vi "CRYStart Editor.vi"(11 "Project Tree reference":refnum<vi>) -> (1 "Steps config.":bool[](array[boolean]))   [LabVIEW 2013]
uses:
  Typedef Control/CRYStart Cluster.ctl
panel:
  in  "Update Display during sequence":bool caption="在运行序列中更新显示步骤"
  in  "Clear measured data at start of sequence":bool caption="在序列开始时清除测试数据"
  in  "Close opened Display at start of sequence":bool caption="在序列开始时关闭打开显示步骤"
  in  "Preload Stimulus":bool caption="预加载激励"
  out "Step Name":string
  in  "Use same Calibration in all subsequences":bool caption="在所有的局部序列使用相同的校准"
  in  "Use same Hardware in all subsequences":bool caption="在所有的局部序列使用相同的硬件"
  in  "Halt on FAIL":bool caption="失败时中断"
  in  "Display for confirmation":bool caption="显示确认"
  in  "Cancel button":bool
  in  "OK button":bool
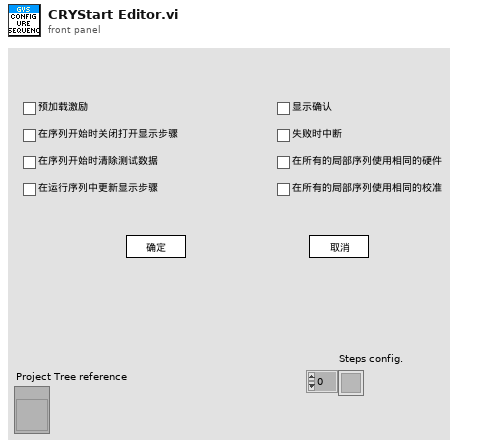
[diagram p1: front panel]
types:
  T1 = typedef "CRYStep.ctl" = cluster{"No.VI":i32, "Category":string, "StepName":string, "Seq setup flattened":string, "Comment":string, "Steps config.":bool[], "Jump config":i32[], "Start":dbl, "Increment":dbl, "Name":string, "Unit":string, "Y data":u16, "Y prefix":string, "Y dB ref":dbl, "Y unit":string, "Repeat State Array":cluster{"Start":dbl, "Increment":dbl, "Count":i32, "Num":i32}[]}
  T2 = typedef "CRYStart Cluster.ctl" = cluster{"SequenceName":string, "Preload Stimulus":bool, "CloseOpenedDisplay":bool, "ClearMeasuredData":bool, "UpdateDisplayDuringRun":bool, "DisplayForConfirmation":bool, "HaltOnFail":bool, "UseSameHardware":bool, "UseSameCalibration":bool}
  T3 = cluster{"SourceRowNum":i32, "SourceCount":i32, "TargetRowNum":i32, "bResult":bool, "EditRowNum":i32}
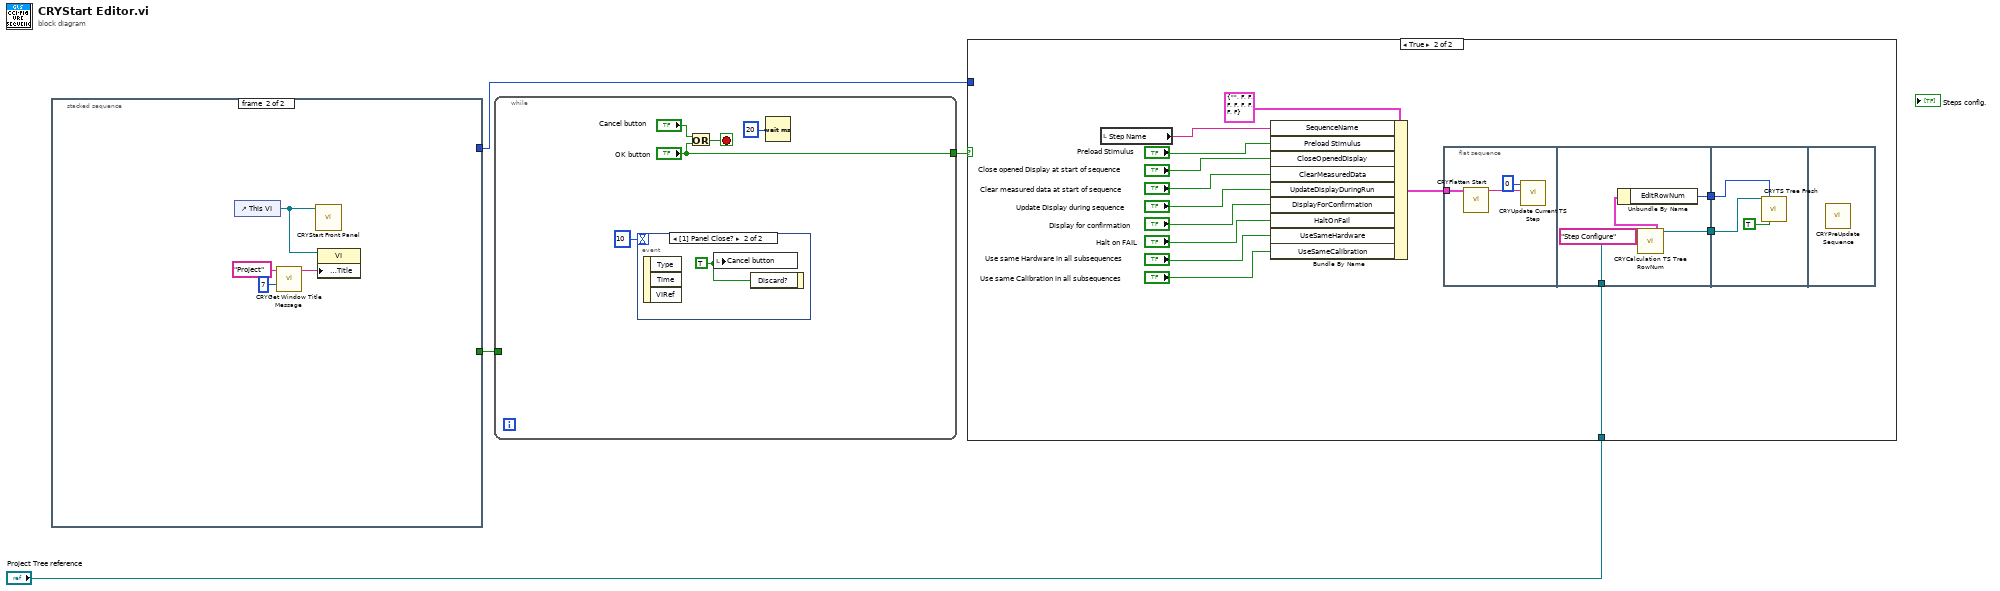
[diagram p0: block diagram]
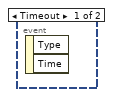
[diagram p2: hidden frame]
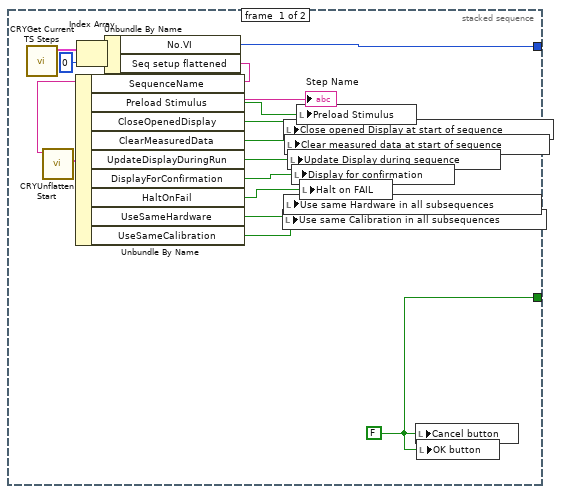
[diagram p4: hidden frame]
diagram:
  n1 = stacked-sequence {
    tunnel: [w20 _] -> w3
    tunnel: [w6 _] -> w2
    frame #0 {
      w20 = FALSE ("Cancel button")
      n2 = call "CRYGet Current TS Steps.vi"() -> ("Steps"=w18:T1[])  [unwired: 1 in, 10 out]
      n3 = Index Array(array=w18, index=0) -> (element=w19:T1)
      n4 = Unbundle By Name(w19) -> ("No.VI"=w6:i32, "Seq setup flattened"=w17:string)
      n5 = call "CRYUnflatten Start.vi"("Unflatten Sequence"=w17) -> ("Sequence Configure"=w16:T2)  [unwired: 8 in, 2 out]
      n6 = Unbundle By Name(w16) -> ("SequenceName"=→"Step Name":string, "Preload Stimulus"=w14:bool, "CloseOpenedDisplay"=w13:bool, "ClearMeasuredData"=w12:bool, "UpdateDisplayDuringRun"=w11:bool, "DisplayForConfirmation"=w10:bool, "HaltOnFail"=w9:bool, "UseSameHardware"=w8:bool, "UseSameCalibration"=w7:bool)
      n7 = local write "Use same Calibration in all subsequences"(w7) -> ()
      n8 = local write "Close opened Display at start of sequence"(w13) -> ()
      n9 = local write "Use same Hardware in all subsequences"(w8) -> ()
      n10 = local write "Clear measured data at start of sequence"(w12) -> ()
      n11 = local write "Update Display during sequence"(w11) -> ()
      n12 = local write "Display for confirmation"(w10) -> ()
      n13 = local write "Preload Stimulus"(w14) -> ()
      n14 = local write "Halt on FAIL"(w9) -> ()
      n15 = local write "Cancel button"(w20) -> ()
      n16 = local write "OK button"(w20) -> ()
    }
    frame #1 {
      n17 = control-ref of="This VI"() -> (w21:refnum<vi>)
      n18 = call "CRYGet Window Title Message.vi"("No"=7, "Kind"="Project") -> ("Multibyte String"=w22:string)  [unwired: 4 in, 5 out]
      n19 = call "CRYStart Front Panel.vi"("Vi Ref"=w21) -> ()  [unwired: 11 in]
      n20 = property class="VI"(reference=w21, "Front Panel.Title"=w22) -> ()  [unwired: 1 in, 2 out]
    }
  }
  n21 = while {
    tunnel: ["OK button"] -> w4
    tunnel: w3 -> [_]
    stop <- w29 stop-if-true
    n22 = event shown="[1] Panel Close?" {
      selector: _ -> [_ _]
      dyn-events: _ -> [_ _]
      timeout: 10 -> [_ _]
      event Timeout {
        n23 = event-data() -> ()  [unwired: 1 in, 2 out]
      }
      event Panel Close? {
        w30 = TRUE ("Discard?")
        n24 = event-data() -> ()  [unwired: 1 in, 3 out]
        n25 = local write "Cancel button"(w30) -> ()
        n26 = event-data("Discard?"=w30) -> ()  [unwired: 1 in, 1 out]
      }
    }
    n27 = Or(x="Cancel button", y="OK button") -> (x .or. y?=w29:bool)
    n28 = Wait (ms)(milliseconds to wait=u32 20) -> ()  [unwired: 1 out]
  }
  n29 = case shown="True" w4 {
    tunnel: w2 -> [_ _]
    tunnel: "Project Tree reference" -> [_ w33]
    frame False {
    }
    frame True {
      n30 = local read "Step Name"() -> (w34:string)
      n31 = Bundle By Name(cluster=T2 {"SequenceName"="", "Preload Stimulus"=FALSE, "CloseOpenedDisplay"=FALSE, "ClearMeasuredData"=FALSE, "UpdateDisplayDuringRun"=FALSE, "DisplayForConfirmation"=FALSE, "HaltOnFail"=FALSE, "UseSameHardware"=FALSE, "UseSameCalibration"=FALSE} ("Sequence Configure"), "SequenceName"=w34, "Preload Stimulus"="Preload Stimulus", "CloseOpenedDisplay"="Close opened Display at start of sequence", "ClearMeasuredData"="Clear measured data at start of sequence", "UpdateDisplayDuringRun"="Update Display during sequence", "DisplayForConfirmation"="Display for confirmation", "HaltOnFail"="Halt on FAIL", "UseSameHardware"="Use same Hardware in all subsequences", "UseSameCalibration"="Use same Calibration in all subsequences") -> (w35:T2)
      n32 = flat-sequence {
        tunnel: w35 -> [w47]
        tunnel: w33 -> [w50]
        tunnel: [w49] -> w32
        tunnel: [w48] -> w31
        tunnel: w32 -> [w54]
        tunnel: w31 -> [w53]
        frame #0 {
          n33 = call "CRYFlatten Start.vi"("Start"=w47) -> ("Start flattened"=w45:string)  [unwired: 10 in]
          n34 = call "CRYUpdate Current TS Step.vi"("setup flattened"=w45, "step index"=0) -> ()  [unwired: 10 in]
        }
        frame #1 {
          n35 = call "CRYCalculation TS Tree RowNum.vi"("Tree Task SequenceIn"=w50, "sOption"="Step Configure") -> ("DispInfo Cluster Out"=w52:T3, "Tree Task Sequence Out"=w49:refnum<vi>)  [unwired: 7 in, 5 out]
          n36 = Unbundle By Name(w52) -> ("EditRowNum"=w48:i32)
        }
        frame #2 {
          n37 = call "CRYTS Tree Fresh.vi"("SequenceTree"=w54, "Edit Index"=w53, "Is Refresh?"=TRUE) -> ()  [unwired: 12 in, 1 out]
        }
        frame #3 {
          n38 = call "CRYPreUpdate Sequence.vi"() -> ()  [unwired: 16 in]
        }
      }
    }
  }
